vi "IOScan_PeriodUnitStrings.vi"() -> (3 "Unit Strings":string[](array[string]))   [LabVIEW 2016]
uses:
  <resource>/dialog/TargetPreferencePages/IOScan_SubVIs/IOScan_TimeUnit.ctl
panel:
  in  "Scan Period Units":T1 items=["us", "ms", "secs"]
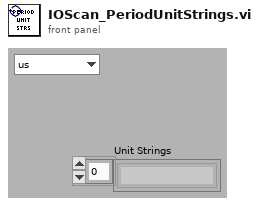
[diagram p1: front panel]
types:
  T1 = typedef "IOScan_TimeUnit.ctl" = u16
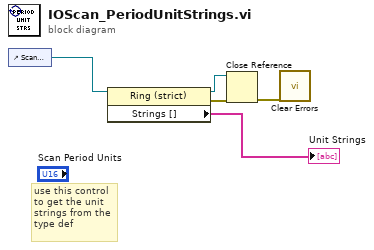
[diagram p0: block diagram]
diagram:
  # "use this control to get the unit strings from the type def"
  n1 = control-ref of="Scan Period Units"() -> (w2:refnum<vi>)
  n2 = property class="Ring (strict)"(reference=w2) -> (reference out=w5:refnum<vi>, error out=w4:errorcluster, "Strings []"=→"Unit Strings":string[])  [unwired: 1 in]
  n3 = Close Reference(reference=w5, error in (no error)=w4) -> (error out=w1:errorcluster)
  n4 = call <vilib>:"Clear Errors.vi"("error in (no error)"=w1) -> ()  [unwired: 5 in, 2 out]
